vi "Get Headers.Text.vi"(8 "error in (no error)":errorcluster, 11 "xwpfDocument in":refnum<class "xwpfDocument.lvclass">) -> (0 "error out":errorcluster, 2 "Headers.Text":string[](array[string]), 3 "xwpfDocument out":refnum<class "xwpfDocument.lvclass">)   [LabVIEW 2017, in "Word_Specific.lvlib" / "xwpfDocument.lvclass"]
uses:
  xwpfDocument.lvclass
  xwpfDocument.lvclass/xwpfDocument.ctl
  xwpfHeader_Footer/Get Paragraphs.Text.vi
  xwpfHeader_Footer/xwpfHeader_Footer.lvclass
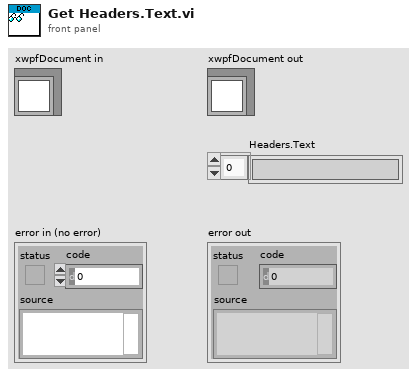
[diagram p1: front panel]
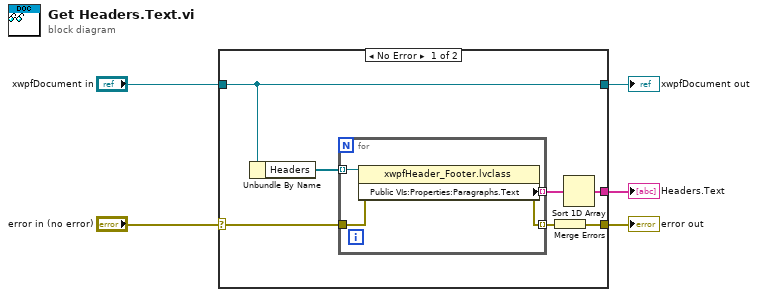
[diagram p0: block diagram]
diagram:
  n1 = case shown="No Error" "error in (no error)" {
    selector: "error in (no error)" -> [w7 w17]
    tunnel: [w8 w17] -> w4
    tunnel: [w12 w18] -> w2
    tunnel: "xwpfDocument in" -> [w12 w18]
    tunnel: [w6 _] -> w1
    frame No Error {
      n2 = Unbundle By Name(w12) -> ("Headers"=w11:refnum<class "xwpfHeader_Footer.lvclass">[])
      n3 = for {
        tunnel: w11 -> [w16] mode=indexing
        tunnel: [w15] -> w10 mode=indexing
        tunnel: [w14] -> w9 mode=indexing
        tunnel: w7 -> [w13]
        n4 = property class="xwpfHeader_Footer.lvclass"(reference=w16, error in=w13) -> (error out=w14:errorcluster, "Public VIs:Properties:Paragraphs.Text"=w15:string)  [unwired: 1 out]
      }
      n5 = Merge Errors(w9) -> (w8:errorcluster)
      n6 = Sort 1D Array(array=w10) -> (sorted array=w6:string[])
    }
    frame Error {
    }
  }
  "error out" <- w4
  "xwpfDocument out" <- w2
  "Headers.Text" <- w1
